vi "gen_syg_u.vi"(0 "Amplituda":dbl, 1 "czestotliwosc":dbl, 2 "Offset":dbl, 3 "rodzaj":T1(ring), 4 "probka":i32) -> (5 "Wyjscie":dbl(graph))   [LabVIEW 2023]
doc: "Generator punkt po punkcie. Pozwala na wybranie sygnalow: sinusoidalnego, prostokatnego, trojkatnego, piloksztaltnego."
uses:
  <vilib>/ptbypt/NI_PtbyPt.lvlib
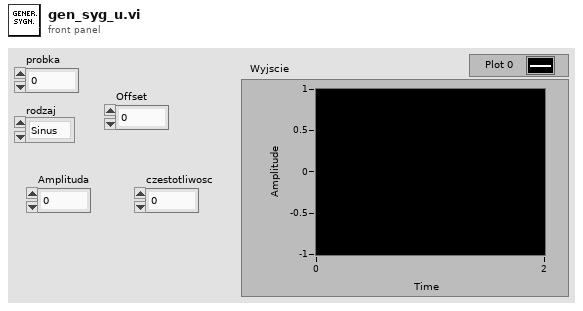
[diagram p1: front panel]
types:
  T1 = enum16{"Sinus", "Rectangle", "Triangle", "Sawthooth"}
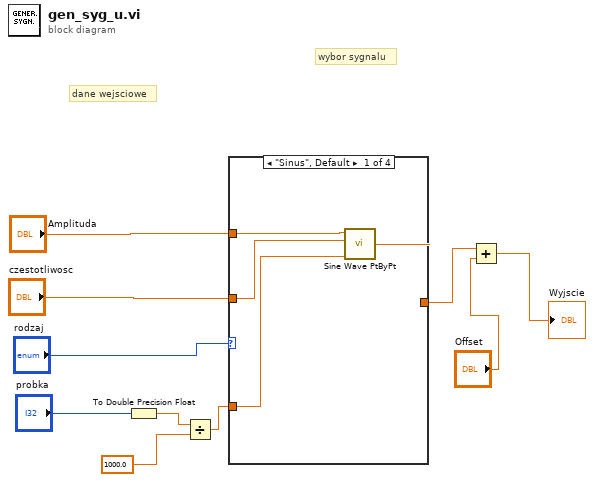
[diagram p0: block diagram]
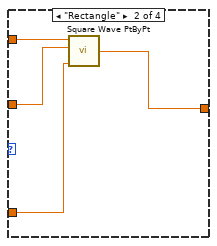
[diagram p2: hidden frame]
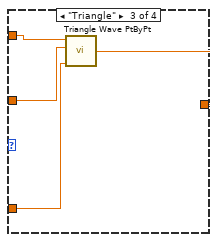
[diagram p3: hidden frame]
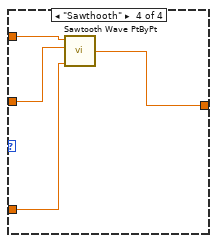
[diagram p4: hidden frame]
diagram:
  # "wybor sygnalu"
  # "dane wejsciowe"
  n1 = To Double Precision Float(number="probka") -> (double precision float=w1:dbl)
  n2 = Divide(x=w1, y=1000.0) -> (x/y=w7:dbl)
  n3 = case shown="\"Sinus\", Default" "rodzaj" {
    tunnel: w7 -> [w14 w17 w21 w25]
    tunnel: "czestotliwosc" -> [w13 w18 w22 w26]
    tunnel: [w12 w16 w20 w24] -> w3
    tunnel: "Amplituda" -> [w11 w15 w19 w23]
    frame "Sinus", Default {
      n4 = call <vilib>:"Sine Wave PtByPt.vi"("time"=w14, "frequency"=w13, "amplitude"=w11) -> ("sine wave"=w12:dbl)  [unwired: 1 in]
    }
    frame "Rectangle" {
      n5 = call <vilib>:"Square Wave PtByPt.vi"("amplitude"=w15, "frequency"=w18, "time"=w17) -> ("square wave"=w16:dbl)  [unwired: 2 in]
    }
    frame "Triangle" {
      n6 = call <vilib>:"Triangle Wave PtByPt.vi"("time"=w21, "frequency"=w22, "amplitude"=w19) -> ("triangle wave"=w20:dbl)  [unwired: 1 in]
    }
    frame "Sawthooth" {
      n7 = call <vilib>:"Sawtooth Wave PtByPt.vi"("time"=w25, "frequency"=w26, "amplitude"=w23) -> ("sawtooth wave"=w24:dbl)  [unwired: 1 in]
    }
  }
  n8 = Add(x=w3, y="Offset") -> (x+y=→"Wyjscie":dbl)
